vi "Find_String.vi"(8 "error in":errorcluster, 10 "String to find":string="OPEN", 11 "Input string":string) -> (0 "error out":errorcluster, 1 "after substring":string, 2 "before substring":string, 3 "Found?":bool)   [LabVIEW 2023]
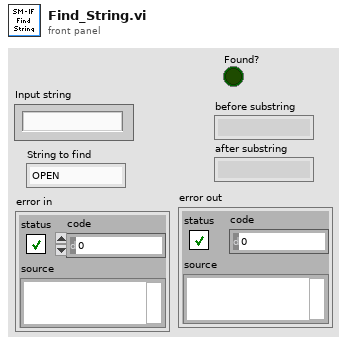
[diagram p1: front panel]
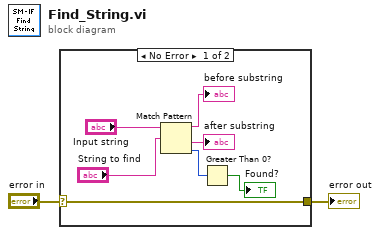
[diagram p0: block diagram]
diagram:
  n1 = case shown="No Error" "error in" {
    selector: "error in" -> [w5 w10]
    tunnel: [w5 w10] -> w1
    frame No Error {
      n2 = Match Pattern(string="Input string", regular expression="String to find") -> (before substring=→"before substring":string, after substring=→"after substring":string, offset past match=w7:i32)  [unwired: 1 in, 1 out]
      n3 = Greater Than 0?(x=w7) -> (x > 0?=→"Found?":bool)
    }
    frame Error {
    }
  }
  "error out" <- w1
